vi "test get channel group.vi"() -> ()   [LabVIEW 2013, in "TBM Tests.lvlib"]
uses:
  TBM Tests.lvlib
  channel/channel classification.ctl
  channel/TBM channel.lvclass
  <vilib>/NI/Tag Bus/dictionary/data dictionary.lvclass
panel:
  out "lookup ok":bool
  out "count ok":bool
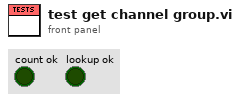
[diagram p1: front panel]
types:
  T1 = typedef "TBM channel.lvclass/channel classification.ctl" = enum16{"input data", "output data", "processing parameter", "processing result"}
  T2 = typedef "tag bus.lvlib/tag descriptor.lvclass/Data Type.ctl" = enum16{"Double", "Single", "I64", "I32", "I16", "I8", "U64", "U32", "U16", "U8", "Boolean", "String", "Array of Double", "Array of Single", "Array of I64", "Array of I32", "Array of I16", "Array of I8", "Array of U64", "Array of U32", "Array of U16", "Array of U8", "Array of Boolean", "Array of String"}
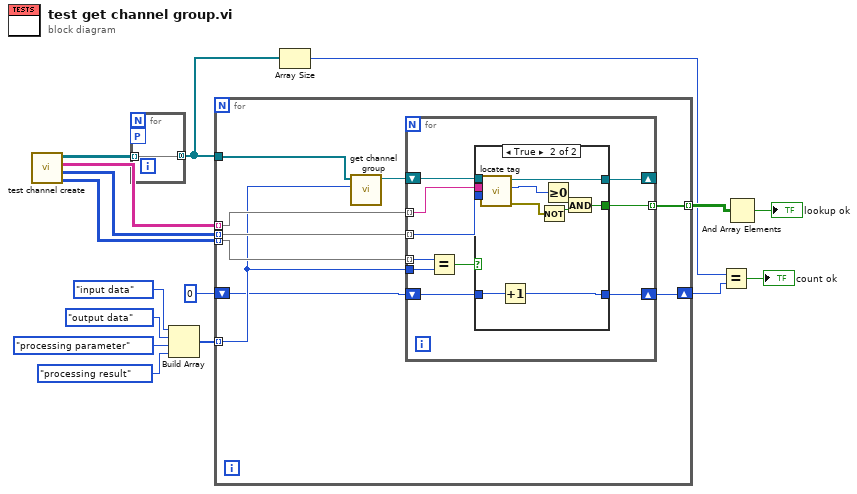
[diagram p0: block diagram]
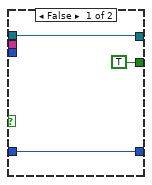
[diagram p2: hidden frame]
diagram:
  n1 = call "test channel create.vi"() -> ("dirs"=w9:T1[][], "types"=w8:T2[][], "names"=w10:string[][], "chans"=w11:refnum<class "TBM channel.lvclass">[][])  [unwired: 8 in]
  n2 = for {
    tunnel: w11 -> [w17] mode=indexing
    tunnel: [w17] -> w6 mode=concatenating
    workers-P: _ -> [_]
  }
  n3 = Build Array(channel_classification."input data" ("channel classification"), channel_classification."output data" ("channel classification"), channel_classification."processing parameter" ("channel classification"), channel_classification."processing result" ("channel classification")) -> (w12:T1[])
  n4 = for {
    tunnel: w12 -> [w21] mode=indexing
    tunnel: w6 -> [w26]
    tunnel: w10 -> [w24] mode=indexing
    tunnel: w9 -> [w22] mode=indexing
    tunnel: w8 -> [w23] mode=indexing
    tunnel: [w20] -> w7 mode=indexing
    shift-right: [w18] -> w4
    shift-left: 0 -> [w19]
    n5 = call "get channel group.vi"("channel classification"=w21, "channels"=w26) -> ("dictionary"=w25:refnum<class "data dictionary.lvclass">)  [unwired: 7 in, 2 out]
    n6 = for {
      shift-right: [w35] -> _
      shift-left: w25 -> [w36]
      tunnel: w24 -> [w34] mode=indexing
      tunnel: w23 -> [w33] mode=indexing
      tunnel: [w32] -> w20 mode=indexing
      tunnel: w22 -> [w31] mode=indexing
      tunnel: w21 -> [w30]
      shift-right: [w28] -> w18
      shift-left: w19 -> [w27]
      n7 = Equal?(x=w31, y=w30) -> (x = y?=w29:bool)
      n8 = case shown="True" w29 {
        tunnel: w36 -> [w39 w50]
        tunnel: [w39 w49] -> w35
        tunnel: w34 -> [_ w48]
        tunnel: w33 -> [_ w47]
        tunnel: [TRUE w42] -> w32
        tunnel: [w37 w40] -> w28
        tunnel: w27 -> [w37 w41]
        frame False {
        }
        frame True {
          n9 = call <vilib>:"locate tag.vi"("data type"=w47, "name"=w48, "data dictionary in"=w50) -> ("error out"=w45:errorcluster, "index"=w46:i32, "data dictionary out"=w49:refnum<class "data dictionary.lvclass">)  [unwired: 6 in]
          n10 = Increment(x=w41) -> (x+1=w40:i32)
          n11 = Not(x=w45) -> (.not. x?=w43:bool)
          n12 = Greater Or Equal To 0?(x=w46) -> (x >= 0?=w44:bool)
          n13 = And(x=w44, y=w43) -> (x .and. y?=w42:bool)
        }
      }
    }
  }
  n14 = Array Size(array=w6) -> (size(s)=w3:i32)
  n15 = Equal?(x=w3, y=w4) -> (x = y?=→"count ok":bool)
  n16 = And Array Elements(Boolean array=w7) -> (logical AND=→"lookup ok":bool)
